vi "ReadFreq.vi"(0 "reference in":refnum<class "Frequency_Counter_Base.lvclass">, 5 "error in (no error)":errorcluster) -> (14 "reference in":refnum<class "Frequency_Counter_Base.lvclass">, 16 "Frequency":dbl, 19 "error out":errorcluster)   [LabVIEW 2022 SP3, in "Frequency_Counter_Base.lvlib" / "Frequency_Counter_Base.lvclass"]
uses:
  Frequency_Counter_Base.lvclass
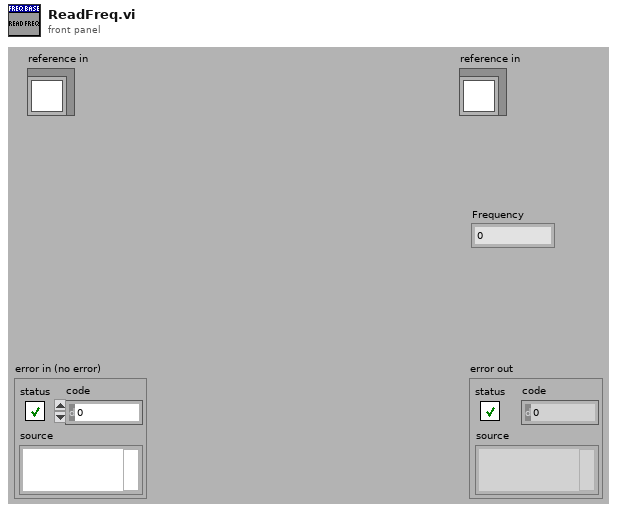
[diagram p1: front panel]
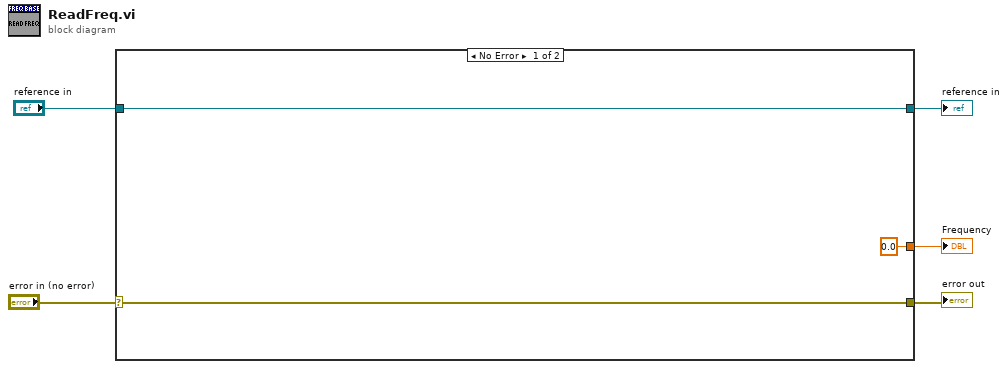
[diagram p0: block diagram]
diagram:
  n1 = case shown="No Error" "error in (no error)" {
    selector: "error in (no error)" -> [w7 w10]
    tunnel: [w7 w10] -> w4
    tunnel: [w8 w9] -> w2
    tunnel: "reference in" -> [w8 w9]
    tunnel: [0.0 _] -> w1
    frame No Error {
    }
    frame Error {
    }
  }
  "error out" <- w4
  "reference in" <- w2
  "Frequency" <- w1
